vi "PropPage_Decoration.vi"() -> (2 "OKtoQuit":bool)   [LabVIEW 2020]
uses:
  7807a0a9-c6b7-4004-97be-31df0e67d86d.vi
  02e82925-0999-4454-9ed4-27f35d04f7b7.vi
  e1568083-ec82-470e-83ca-6b1ad1c59f6f.vi
  833798b8-c358-4a31-9010-3e3d773e8ec5.vi
  b5dd1fea-0a43-4f0c-8a71-3241c64c98eb.vi
  d57ffcc1-9411-4d45-8b31-e92628e0ac75.vi
panel:
  in  "FG Color":u32(colorbox)
  in  "BG Color":u32(colorbox)
  in  "Top":i32
  in  "Left":i32
  in  "Height":u32 step=1
  in  "Width":u32 step=1
  in  "QueueName":string
  in  "Main Ref Array In":refnum<vi>[](array[refnum])
  # "Size"
  # "Position"
  # "Colors"
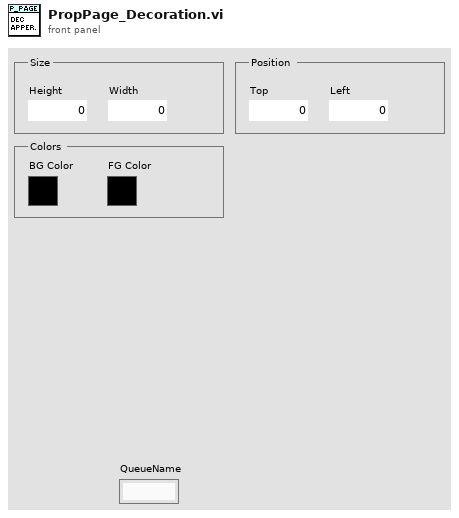
[diagram p1: front panel]
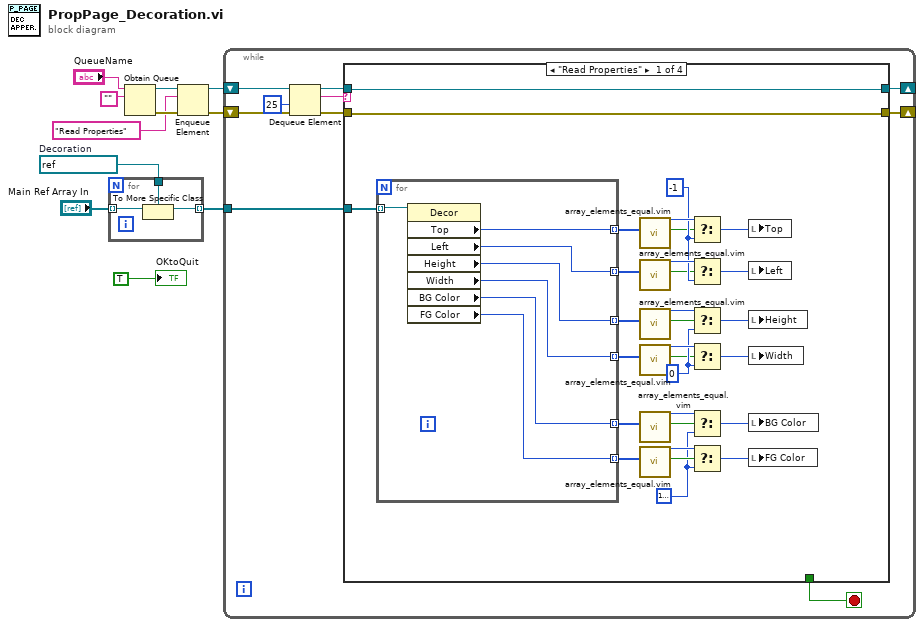
[diagram p0: block diagram]
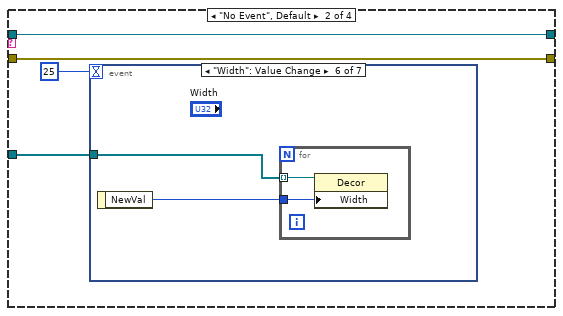
[diagram p2: hidden frame]
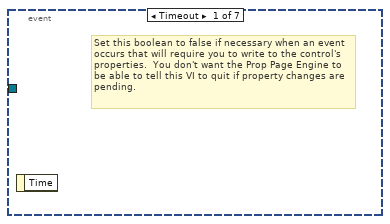
[diagram p3: hidden frame]
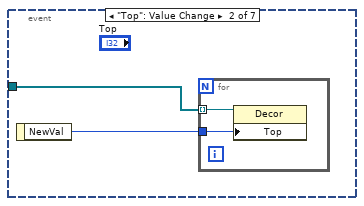
[diagram p4: hidden frame]
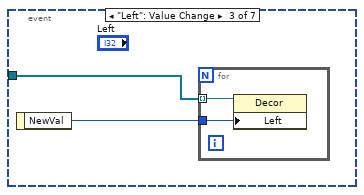
[diagram p5: hidden frame]
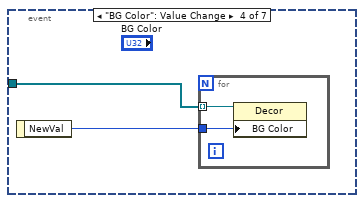
[diagram p6: hidden frame]
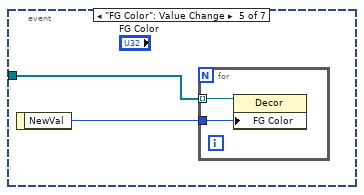
[diagram p7: hidden frame]
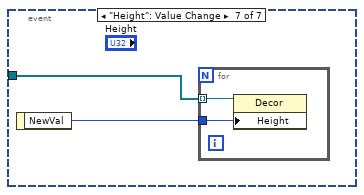
[diagram p8: hidden frame]
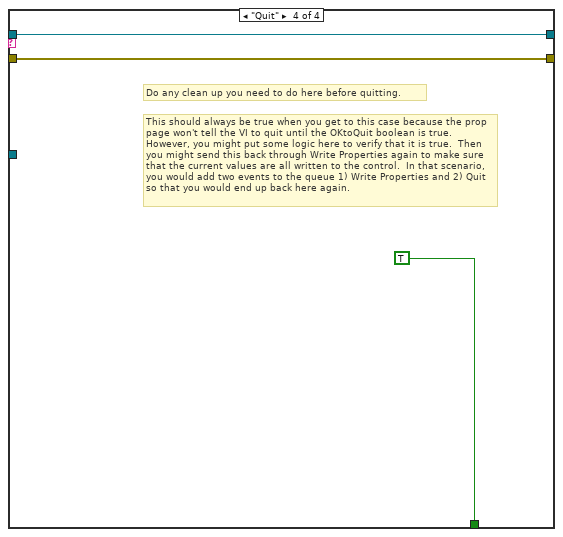
[diagram p10: hidden frame]
diagram:
  w5 = refnum<vi> refnum  # Decoration
  n1 = for {
    tunnel: w5 -> [w14]
    tunnel: "Main Ref Array In" -> [w13] mode=indexing
    tunnel: [w12] -> w3 mode=indexing
    n2 = To More Specific Class(target class=w14, reference=w13) -> (specific class reference=w12:refnum<vi>)  [unwired: 1 in, 1 out]
  }
  n3 = Obtain Queue(name (unnamed)="QueueName", element data type="") -> (queue out=w11:refnum<queue>, error out=w10:errorcluster)  [unwired: 3 in, 1 out]
  n4 = Enqueue Element(queue=w11, element="Read Properties", error in (no error)=w10) -> (queue out=w7:refnum<queue>, error out=w8:errorcluster)  [unwired: 1 in, 1 out]
  n5 = while {
    shift-right: [w21] -> _
    shift-left: w7 -> [w24]
    shift-right: [w20] -> _
    shift-left: w8 -> [w23]
    tunnel: w3 -> [w15]
    stop <- w16 stop-if-true
    n6 = Dequeue Element(queue=w24, timeout in ms (-1)=25, error in (no error)=w23) -> (queue out=w18:refnum<queue>, element=w22:string, error out=w19:errorcluster)  [unwired: 1 out]
    n7 = case shown="\"Read Properties\"" w22 {
      tunnel: [w52 w63 w92 w95] -> w21
      tunnel: [w54 w62 w91 w94] -> w20
      tunnel: w19 -> [w54 w62 w91 w94]
      tunnel: w18 -> [w52 w63 w92 w95]
      tunnel: [_ _ TRUE TRUE] -> w16
      tunnel: w15 -> [w53 w64 _ _]
      frame "Read Properties" {
        w27 = u32 16777216
        w42 = u32 0 ("f")
        w47 = -1 ("f")
        n8 = for {
          tunnel: w53 -> [w61] mode=indexing
          tunnel: [w60] -> w39 mode=indexing
          tunnel: [w59] -> w37 mode=indexing
          tunnel: [w58] -> w35 mode=indexing
          tunnel: [w57] -> w33 mode=indexing
          tunnel: [w56] -> w31 mode=indexing
          tunnel: [w55] -> w29 mode=indexing
          n9 = property class="Decor"(reference=w61) -> ("Top"=w60:i32, "Left"=w59:i32, "Height"=w58:u32, "Width"=w57:u32, "BG Color"=w56:u32, "FG Color"=w55:u32)  [unwired: 1 in, 2 out]
        }
        n10 = call "array_elements_equal.vim"("array"=w39) -> ("elements equal"=w38:bool, "element"=w51:i32)  [unwired: 9 in]
        n11 = call "array_elements_equal.vim"("array"=w37) -> ("elements equal"=w36:bool, "element"=w50:i32)  [unwired: 9 in]
        n12 = call "array_elements_equal.vim"("array"=w35) -> ("elements equal"=w34:bool, "element"=w46:u32)  [unwired: 9 in]
        n13 = call "array_elements_equal.vim"("array"=w33) -> ("elements equal"=w32:bool, "element"=w44:u32)  [unwired: 9 in]
        n14 = call "array_elements_equal.vim"("array"=w31) -> ("elements equal"=w30:bool, "element"=w40:u32)  [unwired: 9 in]
        n15 = call "array_elements_equal.vim"("array"=w29) -> ("elements equal"=w28:bool, "element"=w41:u32)  [unwired: 9 in]
        n16 = Select(t=w51, s=w38, f=w47) -> (s? t:f=w48:i32)
        n17 = Select(t=w50, s=w36, f=w47) -> (s? t:f=w49:i32)
        n18 = Select(t=w46, s=w34, f=w42) -> (s? t:f=w45:u32)
        n19 = Select(t=w44, s=w32, f=w42) -> (s? t:f=w43:u32)
        n20 = Select(t=w40, s=w30, f=w27) -> (s? t:f=w25:u32)
        n21 = Select(t=w41, s=w28, f=w27) -> (s? t:f=w26:u32)
        n22 = local write "Top"(w48) -> ()
        n23 = local write "Left"(w49) -> ()
        n24 = local write "Height"(w45) -> ()
        n25 = local write "Width"(w43) -> ()
        n26 = local write "BG Color"(w25) -> ()
        n27 = local write "FG Color"(w26) -> ()
      }
      frame "No Event", Default {
        n28 = event shown="[5] \"Width\": Value Change" {
          selector: _ -> [_ _ _ _ _ _ _]
          dyn-events: _ -> [_ _ _ _ _ _ _]
          timeout: 25 -> [_ _ _ _ _ _ _]
          tunnel: w64 -> [_ w67 w71 w75 w79 w83 w87]
          event Timeout {
            # "Set this boolean to false if necessary when an event occurs that will require you to write to the control's properties.  You don't want the Prop Page Engine to be able to tell this VI to quit if property changes are pending."
            n29 = event-data() -> ()  [unwired: 1 in, 1 out]
          }
          event "Top": Value Change {
            n30 = event-data() -> ("NewVal"=w66:i32)  [unwired: 1 in]
            n31 = for {
              tunnel: w66 -> [w69]
              tunnel: w67 -> [w68] mode=indexing
              n32 = property class="Decor"(reference=w68, "Top"=w69) -> ()  [unwired: 1 in, 2 out]
            }
          }
          event "Left": Value Change {
            n33 = event-data() -> ("NewVal"=w70:i32)  [unwired: 1 in]
            n34 = for {
              tunnel: w70 -> [w73]
              tunnel: w71 -> [w72] mode=indexing
              n35 = property class="Decor"(reference=w72, "Left"=w73) -> ()  [unwired: 1 in, 2 out]
            }
          }
          event "BG Color": Value Change {
            n36 = event-data() -> ("NewVal"=w74:u32)  [unwired: 1 in]
            n37 = for {
              tunnel: w74 -> [w77]
              tunnel: w75 -> [w76] mode=indexing
              n38 = property class="Decor"(reference=w76, "BG Color"=w77) -> ()  [unwired: 1 in, 2 out]
            }
          }
          event "FG Color": Value Change {
            n39 = event-data() -> ("NewVal"=w78:u32)  [unwired: 1 in]
            n40 = for {
              tunnel: w78 -> [w81]
              tunnel: w79 -> [w80] mode=indexing
              n41 = property class="Decor"(reference=w80, "FG Color"=w81) -> ()  [unwired: 1 in, 2 out]
            }
          }
          event "Width": Value Change {
            n42 = event-data() -> ("NewVal"=w82:u32)  [unwired: 1 in]
            n43 = for {
              tunnel: w82 -> [w85]
              tunnel: w83 -> [w84] mode=indexing
              n44 = property class="Decor"(reference=w84, "Width"=w85) -> ()  [unwired: 1 in, 2 out]
            }
          }
          event "Height": Value Change {
            n45 = event-data() -> ("NewVal"=w86:u32)  [unwired: 1 in]
            n46 = for {
              tunnel: w86 -> [w89]
              tunnel: w87 -> [w88] mode=indexing
              n47 = property class="Decor"(reference=w88, "Height"=w89) -> ()  [unwired: 1 in, 2 out]
            }
          }
        }
      }
      frame "Cancel" {
        # "Any properties or settings that are changed without using property or invoke nodes\nwill not be caught by the undo transaction.  This case will be called when the user\nhits the \"Cancel\" button on the main property page.  So, any settings made should\nreverted programmatically by the developer in this case (note that any settings\ndone using property or invoke nodes will automatically be undone)."
      }
      frame "Quit" {
        # "This should always be true when you get to this case because the prop page won't tell the VI to quit until the OKtoQuit boolean is true.  However, you might put some logic here to verify that it is true.  Then you might send this back through Write Properties again to make sure that the current values are all written to the control.  In that scenario, you would add two events to the queue 1) Write Properties and 2) Quit so that you would end up back here again."
        # "Do any clean up you need to do here before quitting."
      }
    }
  }
  "OKtoQuit" <- TRUE
